vi "Solve2.vi"(8 "Error In":errorcluster, 11 "object in":refnum<class "2024_19.lvclass">) -> (0 "Error Out":errorcluster, 2 "Result":u64, 3 "object out":refnum<class "2024_19.lvclass">)   [LabVIEW 2023, in "2024_19.lvclass"]
uses:
  2024_19.lvclass
  2024_19.lvclass/2024_19.ctl
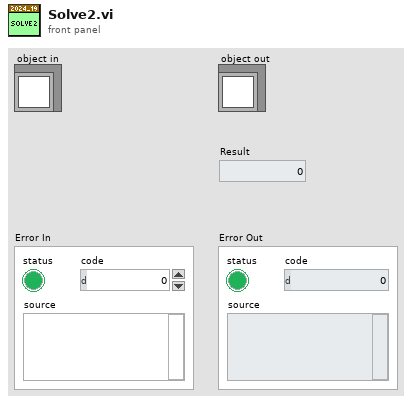
[diagram p1: front panel]
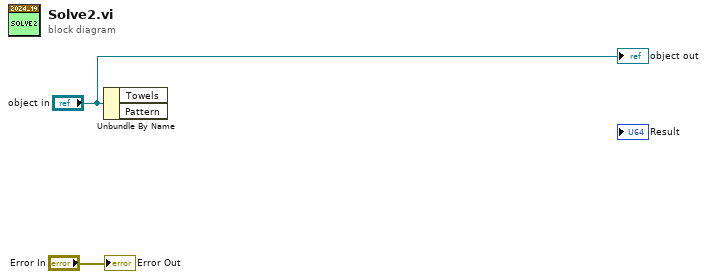
[diagram p0: block diagram]
diagram:
  n1 = Unbundle By Name("object in") -> ()  [unwired: 2 out]
  "Error Out" <- "Error In"
  "object out" <- "object in"
